vi "Create GUI element.vi"(8 "error in (no error)":errorcluster, 11 "Schedule in":refnum<class "Schedule.lvclass">) -> (0 "error out":errorcluster, 2 "Array of Runs":T1 {"Number of cycles" min=1}, 3 "Schedule out":refnum<class "Schedule.lvclass">)   [LabVIEW 2020, in "CIRCUS_uServices.lvlib" / "Run Utilities.lvlib" / "Schedule.lvclass"]
uses:
  Schedule.lvclass
  Array of Runs - GUI.ctl
  Cell/Cell - GUI.ctl
  Run Instance/Run Instance - GUI.ctl
  Cell/Schedule Cell.lvclass
  Run Instance/Run Instance.lvclass
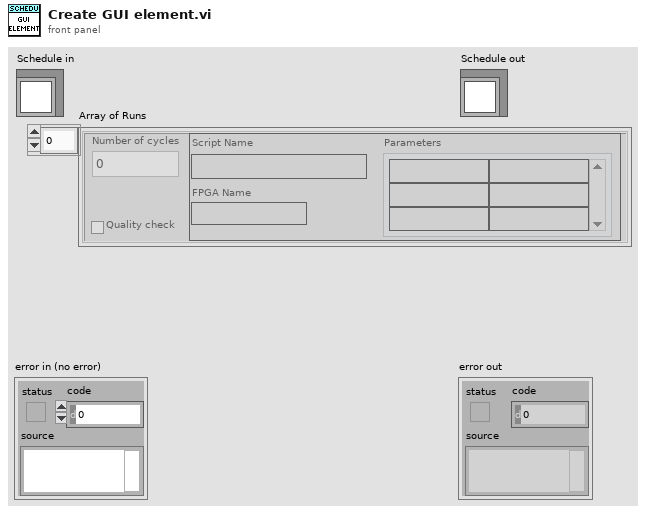
[diagram p1: front panel]
types:
  T1 = typedef "CIRCUS_uServices.lvlib/Run Utilities.lvlib/Schedule.lvclass/Array of Runs - GUI.ctl" = T2[]
  T2 = typedef "CIRCUS_uServices.lvlib/Run Utilities.lvlib/Schedule Cell.lvclass/Cell - GUI.ctl" = cluster{"Background Color":u32, "Number of cycles":u32, "Single RUN":T3, "Quality check":bool, "Cell Type":string}
  T3 = typedef "CIRCUS_uServices.lvlib/Run Utilities.lvlib/Run Instance.lvclass/Run Instance - GUI.ctl" = cluster{"Script Name":string, "Parameters":string[][], "FPGA Name":string}
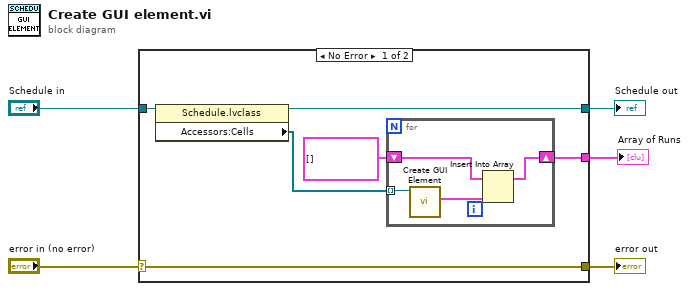
[diagram p0: block diagram]
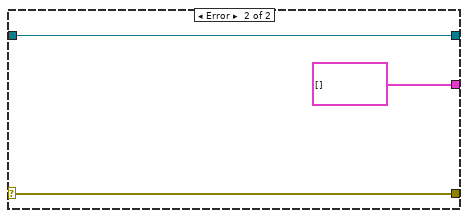
[diagram p2: hidden frame]
diagram:
  n1 = case shown="No Error" "error in (no error)" {
    selector: "error in (no error)" -> [w10 w18]
    tunnel: [w10 w18] -> w4
    tunnel: [w9 w17] -> w2
    tunnel: "Schedule in" -> [w11 w17]
    tunnel: [w6 T1 [] ("Array of Runs")] -> w1
    frame No Error {
      n2 = property class="Schedule.lvclass"(reference=w11) -> (reference out=w9:refnum<class "Schedule.lvclass">, "Accessors:Cells"=w7:refnum<class "Schedule Cell.lvclass">[])  [unwired: 1 in, 1 out]
      n3 = for {
        shift-right: [w14] -> w6
        shift-left: T1 [] ("Array of Runs") -> [w13]
        tunnel: w7 -> [w15] mode=indexing
        n4 = call-dynamic "Create GUI Element.vi"("Schedule Cell in"=w15) -> ("RUN properties"=w12:T2)  [unwired: 8 in, 2 out]
        n5 = Insert Into Array(array=w13, new element=w12) -> (w14:T1)  [unwired: 1 in]
      }
    }
    frame Error {
    }
  }
  "error out" <- w4
  "Schedule out" <- w2
  "Array of Runs" <- w1
